vi "CIPC Channel Errors Core.vi"(8 "error in (no error)":errorcluster, 10 "String to Append":string, 11 "Error":T1) -> (0 "error out":errorcluster)   [LabVIEW 2021, in "CIF_CIPC_Chn.lvclass"]
uses:
  CIF_CIPC_Chn.lvclass
  CIF_CIPC_Chn.lvclass/CIF_CIPC_Chn.ctl
  <vilib>/CIF Foundation/CIF Utilities/Errors/Errors_CIF_U.lvlib
  Typedef/CIPC Channel Error.ctl
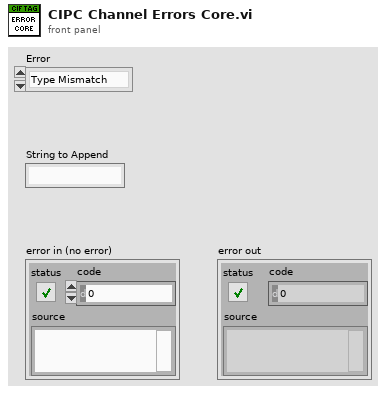
[diagram p1: front panel]
types:
  T1 = typedef "CIF_CIPC_Chn.lvclass/CIPC Channel Error.ctl" = enum16{"Type Mismatch"}
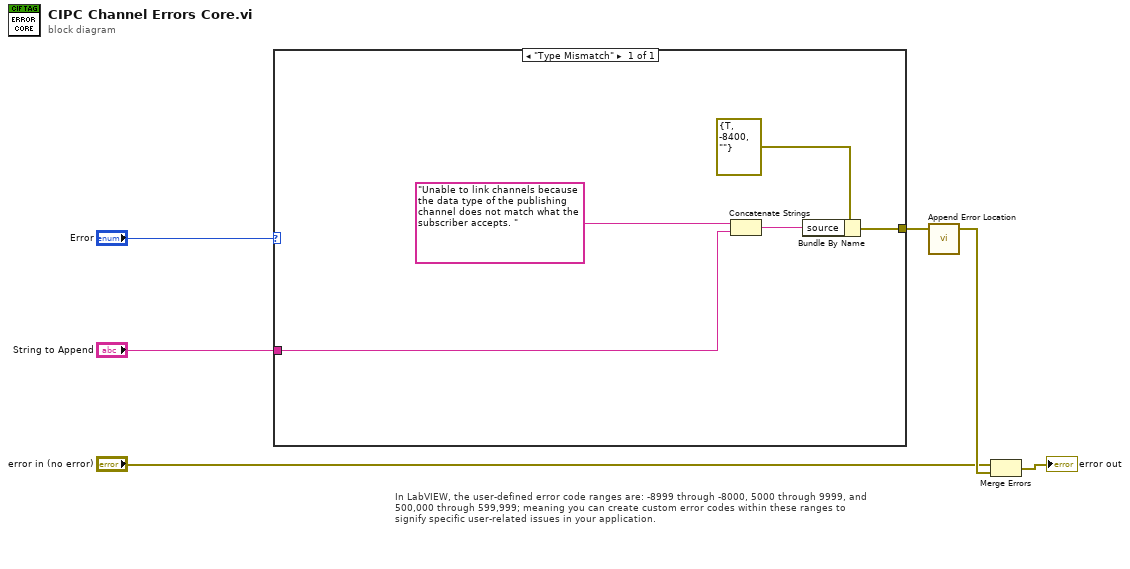
[diagram p0: block diagram]
diagram:
  # "In LabVIEW, the user-defined error code ranges are: -8999 through -8000, 5000 through 9999, and 500,000 through 599,999; meaning you can create custom error codes within these ranges to signify specific user-related issues in your application."
  n1 = case shown="\"Type Mismatch\"" "Error" {
    tunnel: "String to Append" -> [w7]
    tunnel: [w10] -> w5
    frame "Type Mismatch" {
      n2 = Concatenate Strings("Unable to link channels because the data type of the publishing channel does not match what the subscriber accepts. " ("source"), w7) -> (w8:string)
      n3 = Bundle By Name(cluster=errorcluster {"status"=TRUE, "code"=-8400, "source"=""} ("Invalid ID"), "source"=w8) -> (w10:errorcluster)
    }
  }
  n4 = call <vilib>:"Append Error Location.vi"("error in (no error)"=w5) -> ("error out"=w6:errorcluster)  [unwired: 4 in]
  n5 = Merge Errors("error in (no error)", w6) -> (→"error out":errorcluster)
